vi "Read All Noise Measurement.vi"(0 "VISA resource name":refnum<visa-resource-name>, 5 "Maximum Time (10000ms)":u32=10000, 7 "Query Level (0: Zero)":i32(ring) items=["Zero", "One"], 11 "error in (no error)":errorcluster) -> (1 "TI":T1, 2 "RN":T1, 3 "DI":T1, 4 "VISA resource name out":refnum<visa-resource-name>, 6 "ISI":T1, 8 "Misc":T3, 12 "PI":T2, 13 "ABUI":T1, 14 "BUI":T1, 15 "error out":errorcluster)   [LabVIEW 2013, in "Agilent 90000 Series.lvlib"]
doc: "Reads all the RJDJ measurements. It initiates, waits for the acquisition to finish and returns the results of the RJDJ measurement."
uses:
  Agilent 90000 Series.lvlib
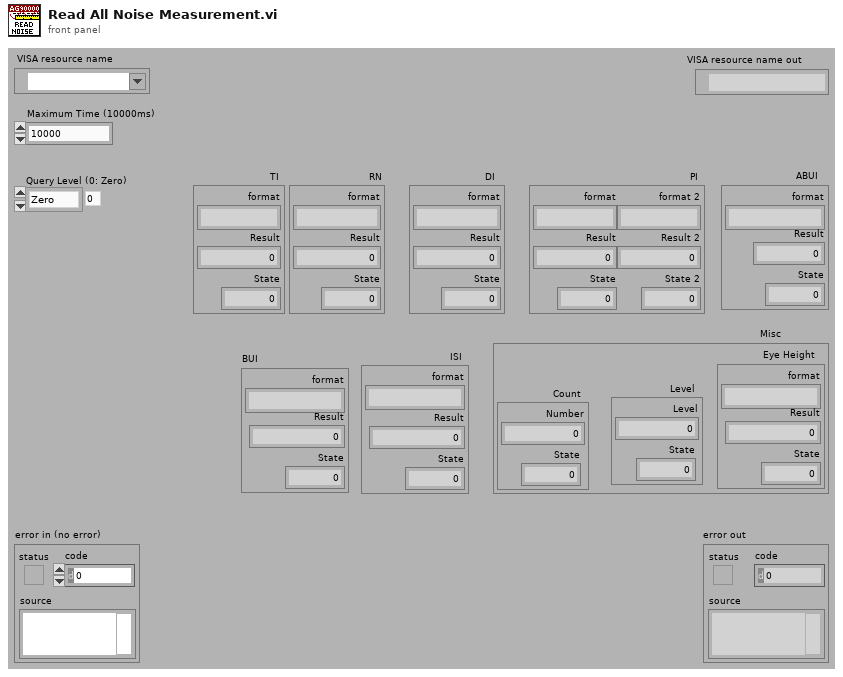
[diagram p1: front panel]
types:
  T1 = cluster{"format":string, "Result":dbl, "State":i32}
  T2 = cluster{"format":string, "Result":dbl, "State":i32, "format 2":string, "Result 2":dbl, "State 2":i32}
  T3 = cluster{"Count":cluster{"Number":dbl, "State":i32}, "Level":cluster{"Level":dbl, "State":i32}, "Eye Height":cluster{"format":string, "Result":dbl, "State":i32}}
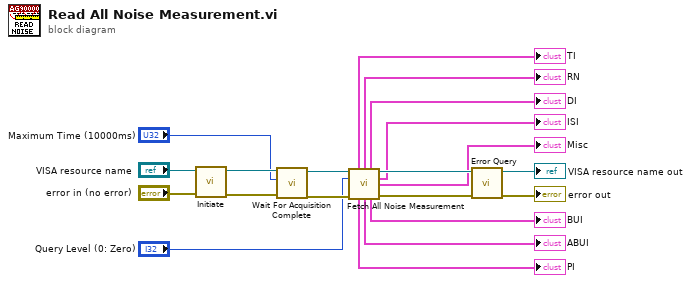
[diagram p0: block diagram]
diagram:
  n1 = call "Initiate.vi"("error in (no error)"="error in (no error)", "VISA resource name"="VISA resource name") -> ("error out"=w17:errorcluster, "VISA resource name out"=w18:refnum<visa-resource-name>)  [unwired: 8 out]
  n2 = call "Wait For Acquisition Complete.vi"("error in (no error)"=w17, "Maximum Time (10000ms)"="Maximum Time (10000ms)", "VISA resource name"=w18) -> ("error out"=w12:errorcluster, "VISA resource name out"=w13:refnum<visa-resource-name>)  [unwired: 7 out]
  n3 = call "Fetch All Noise Measurement.vi"("VISA resource name"=w13, "Query Level (0: Zero)"="Query Level (0: Zero)", "error in (no error)"=w12) -> ("TI"=→"TI":T1, "RN"=→"RN":T1, "DI"=→"DI":T1, "VISA resource name out"=w11:refnum<visa-resource-name>, "ISI"=→"ISI":T1, "Misc"=→"Misc":T3, "PI"=→"PI":T2, "ABUI"=→"ABUI":T1, "BUI"=→"BUI":T1, "error out"=w10:errorcluster)  [unwired: 3 in]
  n4 = call "Error Query.vi"("error in (no error)"=w10, "VISA resource name"=w11) -> ("error out"=→"error out":errorcluster, "VISA resource name out"=→"VISA resource name out":refnum<visa-resource-name>)  [unwired: 2 in, 6 out]
